vi "Chroma 1905x Series Preset Part Number.vi"(2 "error in":T1, 3 "Part Number":string, 4 "inst handle in":refnum<visa-resource-name>) -> (0 "error out":T1, 1 "inst handle out":refnum<visa-resource-name>)   [LabVIEW 2025]
doc: "Chroma\n5 Clock Tower Place Suite 210\nMaynard, MA 01754\nTel: 1 800 253-1230\nTel: 1 877 4 A HIPOT\nFax: 1 978-461-4295\nWebsite: www.Chroma.com"
uses:
  <instrlib>/Chroma 19052/Chroma 19052.lvlib
panel:
  # "Part Number\nNo More than 9 Characters"
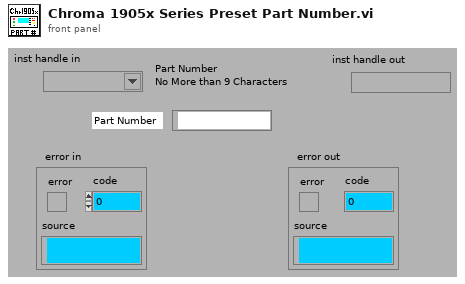
[diagram p1: front panel]
types:
  T1 = cluster{"error":bool, "code":i8, "source":string}
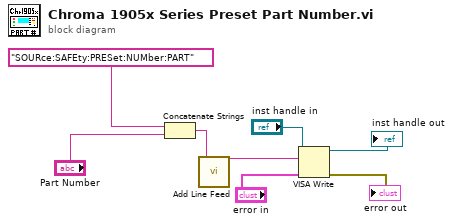
[diagram p0: block diagram]
diagram:
  n1 = Concatenate Strings("SOURce:SAFEty:PRESet:NUMber:PART", "Part Number") -> (w2:string)
  n2 = call <instrlib>:"Add Line Feed.vi"("Cmdstring"=w2) -> ("Concatenated String"=w1:string)
  n3 = VISA Write(VISA resource name="inst handle in", write buffer=w1, error in (no error)="error in") -> (VISA resource name out=→"inst handle out":refnum<visa-resource-name>, error out=→"error out":errorcluster)  [unwired: 1 out]
